vi "SHA_calc_appendsU32.vi"(11 "String length":i32) -> (1 "Second last chunk":string, 2 "Last Chunk":string, 3 "Number of chunks":i32, 5 "Double appends":bool)   [LabVIEW 2012, in "Encryption.lvlib"]
doc: "Calculates the appendices for the last chunks (32-bit).\n\n(c) Ton Plomp, 2011\nTHIS SOFTWARE IS PROVIDED AS IS, AND ANY WARRANTY IS REJECTED"
uses:
  Encryption.lvlib
panel:
  out "x+y":i32
  out "length":i32
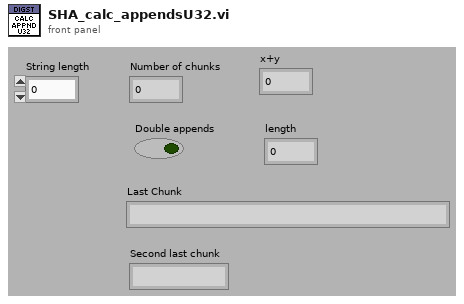
[diagram p1: front panel]
types:
  T1 = enum16{"big-endian, network order", "native, host order", "little-endian"}
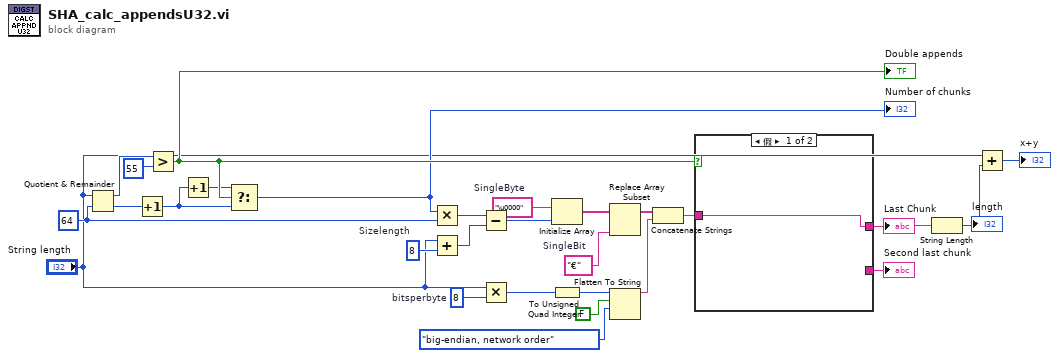
[diagram p0: block diagram]
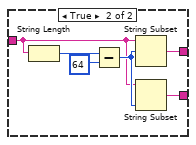
[diagram p2: hidden frame]
diagram:
  w17 = 8  # Sizelength
  w6 = "\u0000"  # SingleByte
  w5 = 8  # bitsperbyte
  w15 = 64 ("y")
  w12 = "€"  # SingleBit
  n1 = Quotient & Remainder(x="String length", y=w15) -> (x-y*floor(x/y)=w22:i32, floor(x/y)=w19:i32)
  n2 = Increment(x=w19) -> (x+1=w24:i32)
  n3 = Greater?(x=w22, y=55) -> (0:w26:bool)
  "Double appends" <- w26
  n4 = Increment(x=w24) -> (x+1=w23:i32)
  n5 = Select(t=w23, s=w26, f=w24) -> (s? t:f=w25:i32)
  "Number of chunks" <- w25
  n6 = Multiply(x=w25, y=w15) -> (x*y=w20:i32)
  n7 = Add(x="String length", y=w17) -> (x+y=w16:i32)
  n8 = Subtract(x=w20, y=w16) -> (x-y=w18:i32)
  n9 = Multiply(x="String length", y=w5) -> (x*y=w7:i32)
  n10 = Initialize Array(w6, w18) -> (w13:string[])
  n11 = To Unsigned Quad Integer(1:w7) -> (0:w8:u64)
  n12 = Replace Array Subset(array=w13, new element=w12) -> (w14:string[])  [unwired: 1 in]
  n13 = Flatten To String(anything=w8, prepend array or string size? (T)=FALSE, byte order (0:big-endian, network order)=T1."big-endian, network order") -> (data string=w11:string)  [unwired: 1 in, 2 out]
  n14 = Concatenate Strings(w14, w11) -> (w27:string)
  n15 = case shown="假" w26 {
    tunnel: w27 -> [w29 w30]
    tunnel: [w29 w35] -> w4
    tunnel: [_ w34] -> w28
    frame False {
    }
    frame True {
      n16 = String Length(string=w30) -> (length=w33:i32)
      n17 = Subtract(x=w33, y=64) -> (x-y=w31:i32)
      n18 = String Subset(string=w30, offset (0)=w31) -> (substring=w35:string)  [unwired: 1 in]
      n19 = String Subset(string=w30, length (rest)=w31) -> (substring=w34:string)  [unwired: 1 in]
    }
  }
  "Last Chunk" <- w4
  "Second last chunk" <- w28
  n20 = String Length(string=w4) -> (length=w2:i32)
  "length" <- w2
  n21 = Add(x="String length", y=w2) -> (x+y=→"x+y":i32)
